vi "ble_discover_handle_table.vi"(6 "Connection Status":T1={"MAC Address"="", "cnx handle"=0, "cnx flags"=0, "Address Type"=125, "Connection Interval (ms)"=125, "Timeout(ms)"=125, "Latency"=0, "bonding handle"=0} {"Address Type" items=["Public", "Random"]}, 8 "error in (no error)":errorcluster, 11 "COM Bluegiga in":refnum<visa-resource-name>) -> (0 "error out":errorcluster, 2 "Handle table":string[][](array[string]), 3 "COM Bluegiga out":refnum<visa-resource-name>)   [LabVIEW 2015]
uses:
  type_def/connection_status_bundle.ctl
  type_def/address_type.ctl
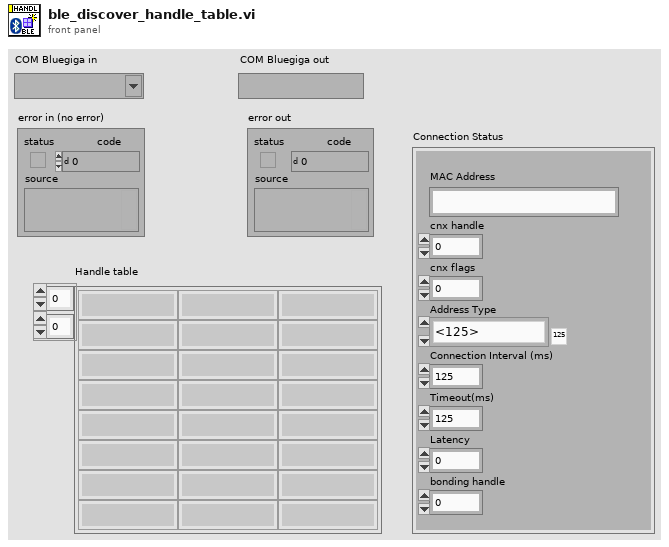
[diagram p1: front panel]
types:
  T1 = typedef "connection_status_bundle.ctl" = cluster{"MAC Address":string, "cnx handle":u8, "cnx flags":u8, "Address Type":T2, "Connection Interval (ms)":u16, "Timeout(ms)":u16, "Latency":u16, "bonding handle":u8}
  T2 = typedef "address_type.ctl" = u8
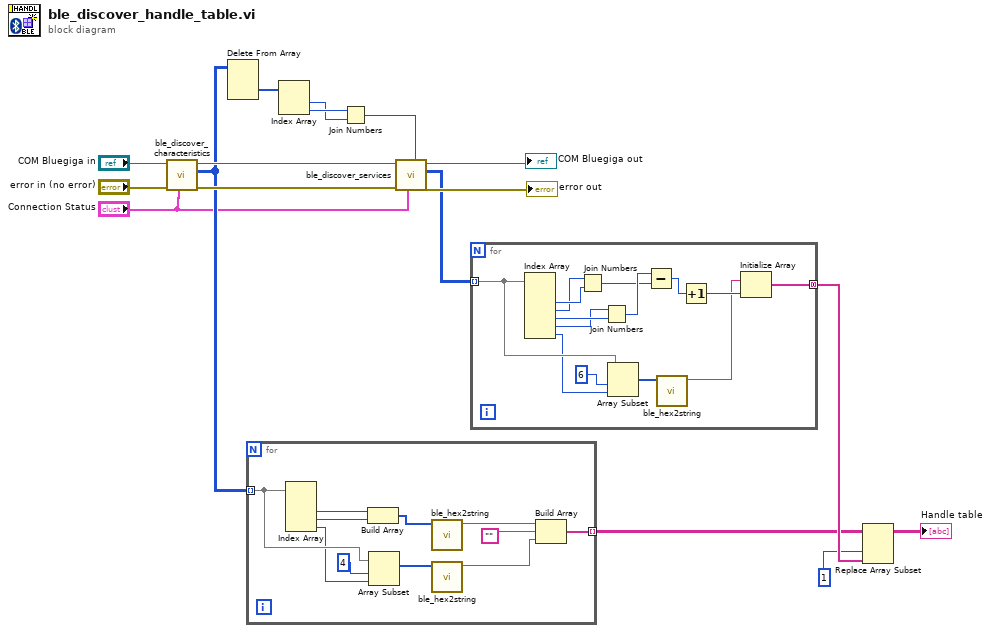
[diagram p0: block diagram]
diagram:
  n1 = call "ble_discover_characteristics.vi"("Connection Status"="Connection Status", "error in (no error)"="error in (no error)", "COM Bluegiga in"="COM Bluegiga in") -> ("error out"=w14:errorcluster, "characteristics_info"=w2:u8[][], "COM Bluegiga out"=w15:refnum<visa-resource-name>)  [unwired: 6 in]
  n2 = Delete From Array(array=w2) -> (deleted portion=w11:u8[])  [unwired: 3 in, 1 out]
  n3 = for {
    tunnel: w2 -> [w28] mode=indexing
    tunnel: [w26] -> w6 mode=indexing
    n4 = Index Array(array=w28) -> (element #2=w23:u8, element #3=w24:u8, element #4=w25:u8)  [unwired: 4 in, 1 out]
    n5 = Build Array(w23, w24) -> (w19:u8[])
    n6 = Array Subset(array=w28, index=4, length=w25) -> (w20:u8[])
    n7 = call "ble_hex2string.vi"("Byte Array IN (index0 LS byte)"=w19) -> ("HEX string OUT"=w18:string)  [unwired: 10 in]
    n8 = call "ble_hex2string.vi"("Byte Array IN (index0 LS byte)"=w20) -> ("HEX string OUT"=w21:string)  [unwired: 10 in]
    n9 = Build Array(w18, "", w21) -> (w26:string[])
  }
  n10 = Index Array(array=w11) -> (element #1=w9:u8, element #2=w10:u8)  [unwired: 2 in]
  n11 = Join Numbers(hi=w10, lo=w9) -> ((hi.lo)=w8:u16)
  n12 = call "ble_discover_services.vi"("Last Handle Number (0xFFFF)"=w8, "Connection Status"="Connection Status", "error in (no error)"=w14, "COM Bluegiga in"=w15) -> ("error out"=→"error out":errorcluster, "service_info"=w3:u8[][], "COM Bluegiga out"=→"COM Bluegiga out":refnum<visa-resource-name>)  [unwired: 5 in]
  n13 = for {
    tunnel: w3 -> [w41] mode=indexing
    tunnel: [w37] -> w7 mode=concatenating
    n14 = Index Array(array=w41) -> (element #2=w32:u8, element #3=w31:u8, element #4=w30:u8, element #5=w29:u8, element #6=w40:u8)  [unwired: 6 in, 1 out]
    n15 = Join Numbers(hi=w31, lo=w32) -> ((hi.lo)=w35:u16)
    n16 = Join Numbers(hi=w29, lo=w30) -> ((hi.lo)=w36:u16)
    n17 = Array Subset(array=w41, index=6, length=w40) -> (w34:u8[])
    n18 = Subtract(x=w36, y=w35) -> (x-y=w42:u16)
    n19 = call "ble_hex2string.vi"("Byte Array IN (index0 LS byte)"=w34) -> ("HEX string OUT"=w33:string)  [unwired: 10 in]
    n20 = Increment(x=w42) -> (x+1=w38:u16)
    n21 = Initialize Array(w33, w38) -> (w37:string[])
  }
  n22 = Replace Array Subset(array=w6, new element=w7, index (col)=1 ("disabled index (col)")) -> (→"Handle table":string[][])  [unwired: 1 in]
